vi "FindChannelByName.vi"(8 "Name":string, 11 "CTRL.Channels in":T1[](array[typedef])) -> (0 "Channel":T1, 1 "Searching":bool, 3 "CTRL.Channels out":T1[](array[typedef]))   [LabVIEW 2016, in "DCM-DSI.lvclass"]
uses:
  DCM-DSI.lvclass
  Channel.ctl
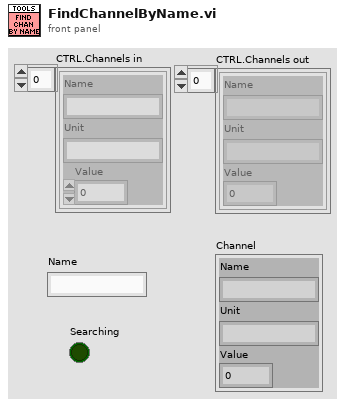
[diagram p1: front panel]
types:
  T1 = typedef "DCM-DSI.lvclass/Channel.ctl" = cluster{"Name":string, "Unit":string, "Value":sgl}
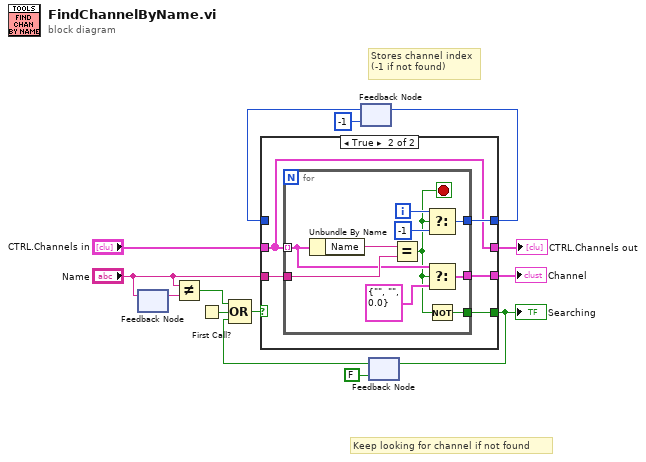
[diagram p0: block diagram]
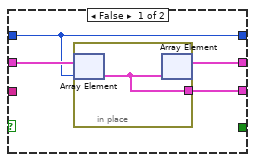
[diagram p2: hidden frame]
diagram:
  # "Stores channel index\n(-1 if not found)"
  # "Keep looking for channel if not found"
  n1 = feedback #1() -> (w10:string)  [unwired: 1 in]
  n2 = feedback-in #1("Name") -> ()
  n3 = Not Equal?(x="Name", y=w10) -> (x != y?=w8:bool)
  n4 = First Call?() -> (First Call?: T/F=w6:bool)
  n5 = feedback #2(-1) -> (w12:i32)
  n6 = feedback #3(FALSE) -> (w3:bool)
  n7 = Compound Arithmetic op=OR(w8, w6, w3) -> (w11:bool)
  n8 = case shown="True" w11 {
    tunnel: "CTRL.Channels in" -> [w18 w21]
    tunnel: "Name" -> [_ w24]
    tunnel: [w15 w23] -> w13
    tunnel: w12 -> [w15 _]
    tunnel: [w17 w22] -> w7
    tunnel: [w16 w21] -> w5
    tunnel: [_ w20] -> w1
    frame False {
      n9 = in-place {
        in-place-border: [w19] -> w17
        n10 = in-place-array #4(w18, w15) -> (w19:T1)
        n11 = in-place-array #4(w19) -> (w16:T1[])  [unwired: 1 out]
      }
    }
    frame True {
      n12 = for {
        tunnel: w21 -> [w29] mode=indexing
        tunnel: w24 -> [w33]
        tunnel: [w30] -> w23
        tunnel: [w28] -> w22
        tunnel: [w25] -> w20
        i -> [w32]
        stop <- w26 stop-if-true
        n13 = Unbundle By Name(w29) -> ("Name"=w34:string)
        n14 = Equal?(x=w34, y=w33) -> (x = y?=w26:bool)
        n15 = Select(t=w32, s=w26, f=-1) -> (s? t:f=w30:i32)
        n16 = Select(t=w29, s=w26, f=T1 {"Name"="", "Unit"="", "Value"=0.0}) -> (s? t:f=w28:T1)
        n17 = Not(x=w26) -> (.not. x?=w25:bool)
      }
    }
  }
  "Channel" <- w7
  "CTRL.Channels out" <- w5
  "Searching" <- w1
  n18 = feedback-in #2(w13) -> ()
  n19 = feedback-in #3(w1) -> ()
